vi "StudentScope - PowerSpectrum.vi"(0 "data":dbl[][](array[numeric]), 1 "Cursor Position":dbl, 5 "Acq Rate (Hz)":dbl) -> (14 "Cursor Freq":string, 15 "Ch0 Amp":string, 16 "Ch1 Amp":string, 17 "Ch0 Freq":string, 18 "Ch1 Freq":string, 19 "Normalized Power Spectrum":cluster{"df":dbl, "df":dbl, "Y":dbl[]}[](array[cluster]))   [LabVIEW 2015]
uses:
  <vilib>/measure/matone.llb/Extract Single Tone Information 1 Chan.vi
  <vilib>/Analysis/NI_AALPro.lvlib
  <vilib>/measure/NI_MAPro.lvlib
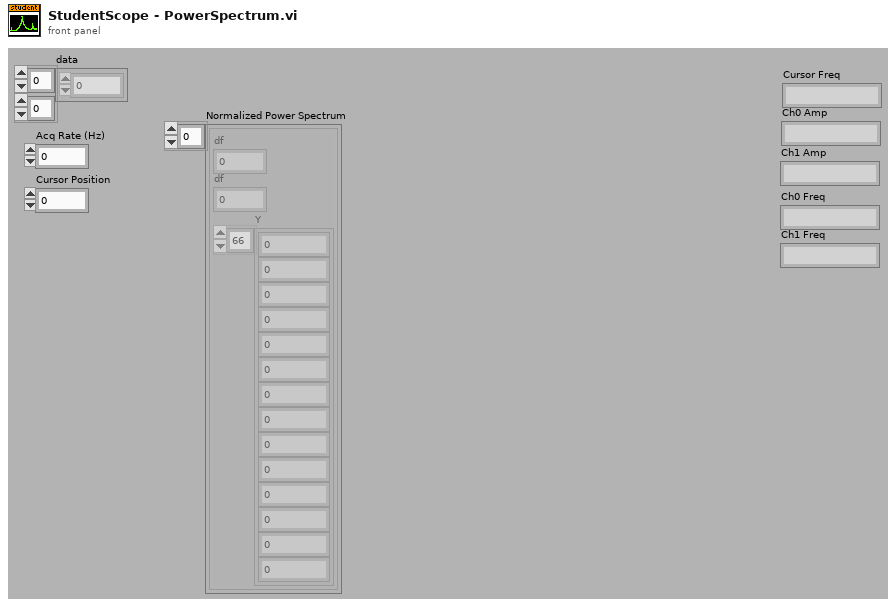
[diagram p1: front panel]
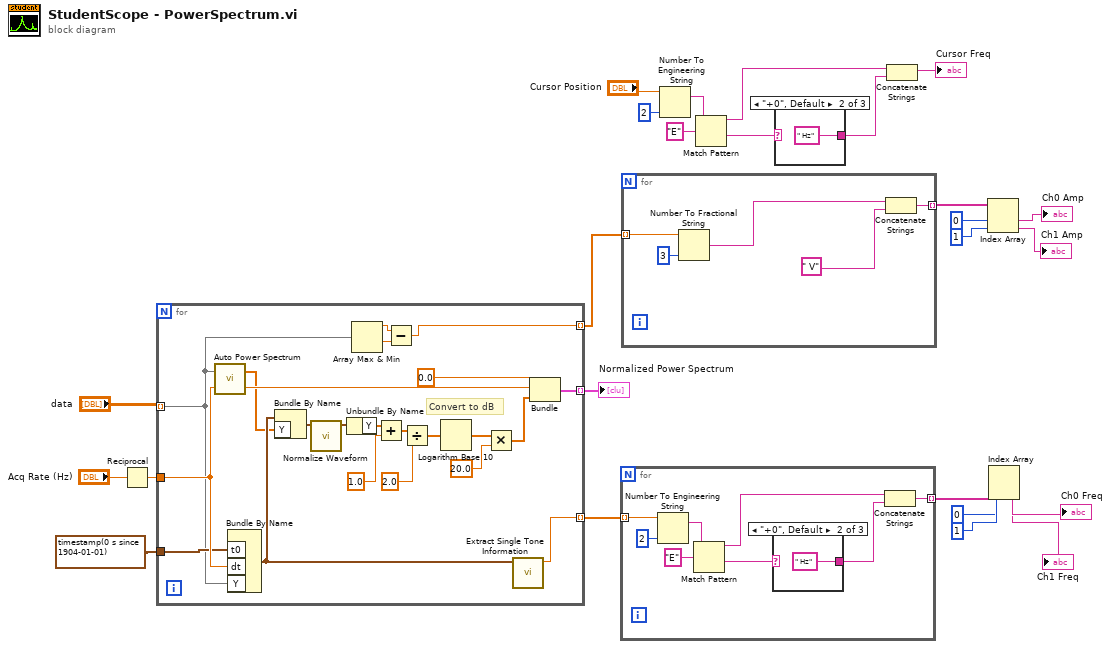
[diagram p0: block diagram]
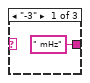
[diagram p2: hidden frame]
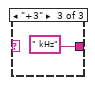
[diagram p3: hidden frame]
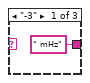
[diagram p4: hidden frame]
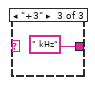
[diagram p5: hidden frame]
diagram:
  n1 = Reciprocal(x="Acq Rate (Hz)") -> (1/x=w23:dbl)
  n2 = for {
    tunnel: "data" -> [w38] mode=indexing
    tunnel: w23 -> [w45]
    tunnel: [w47] -> w20 mode=indexing
    tunnel: [w40] -> w25 mode=indexing
    tunnel: timestamp(0 s since 1904-01-01) ("current time") -> [w39]
    tunnel: [w35] -> w14 mode=indexing
    # "Convert to dB"
    n3 = call <vilib>:"Auto Power Spectrum.vi"("dt"=w45, "Signal (V)"=w38) -> ("df"=w44:dbl, "Power Spectrum (V^2 rms)"=w41:dbl[])
    n4 = Bundle By Name("t0"=w39, "dt"=w45, "Y"=w38) -> (w42:waveform(dbl))  [unwired: 1 in]
    n5 = Bundle By Name(cluster=w42, "Y"=w41) -> (w43:waveform(dbl))
    n6 = call <vilib>:"Normalize Waveform.vi"("waveform in"=w43) -> ("normalized waveform"=w34:waveform(dbl))  [unwired: 7 in, 3 out]
    n7 = Unbundle By Name(w34) -> ("Y"=w31:dbl[])
    n8 = Array Max & Min(array=w38) -> (max value=w37:dbl, min value=w36:dbl)  [unwired: 2 out]
    n9 = Add(x=w31, y=1.0) -> (x+y=w33:dbl[])
    n10 = Subtract(x=w37, y=w36) -> (x-y=w35:dbl)
    n11 = Divide(x=w33, y=2.0) -> (x/y=w27:dbl[])
    n12 = Logarithm Base 10(1:w27) -> (0:w29:dbl[])
    n13 = Multiply(x=w29, y=20.0) -> (x*y=w26:dbl[])
    n14 = call-poly <vilib>:"Extract Single Tone Information.vi"("time signal in"=w42) -> ("detected frequency"=w47:dbl)  [unwired: 5 in, 5 out]
    n15 = Bundle("df"=0.0, "df"=w44, w26) -> (w40:cluster{"df":dbl, "df":dbl, dbl[]})  [unwired: 1 in]
  }
  "Normalized Power Spectrum" <- w25
  n16 = for {
    tunnel: [w49] -> w17 mode=indexing
    tunnel: w20 -> [w48] mode=indexing
    n17 = Number To Engineering String(2:i16 2 ("precision (6)"), 4:w48) -> (0:w55:string)  [unwired: 2 in]
    n18 = Match Pattern(string=w55, regular expression="E" ("string")) -> (before substring=w51:string, after substring=w52:string)  [unwired: 1 in, 2 out]
    n19 = case shown="\"+0\", Default" w52 {
      tunnel: [" mHz" ("string") " Hz" ("string") " kHz" ("string")] -> w50
      frame "-3" {
      }
      frame "+0", Default {
      }
      frame "+3" {
      }
    }
    n20 = Concatenate Strings(w51, w50) -> (w49:string)
  }
  n21 = for {
    tunnel: [w62] -> w11 mode=indexing
    tunnel: w14 -> [w60] mode=indexing
    n22 = Number To Fractional String(number=w60, precision (6)=i16 3) -> (F-format string=w59:string)  [unwired: 2 in]
    n23 = Concatenate Strings(w59, " V" ("string")) -> (w62:string)
  }
  n24 = Number To Engineering String(2:i16 2 ("precision (6)"), 4:"Cursor Position") -> (0:w4:string)  [unwired: 2 in]
  n25 = Match Pattern(string=w4, regular expression="E" ("string")) -> (before substring=w8:string, after substring=w7:string)  [unwired: 1 in, 2 out]
  n26 = case shown="\"+0\", Default" w7 {
    tunnel: [" mHz" ("string") " Hz" ("string") " kHz" ("string")] -> w1
    frame "-3" {
    }
    frame "+0", Default {
    }
    frame "+3" {
    }
  }
  n27 = Concatenate Strings(w8, w1) -> (→"Cursor Freq":string)
  n28 = Index Array(array=w11, index #1=0 ("index"), index #2=1 ("index")) -> (element #1=→"Ch0 Amp":string, element #2=→"Ch1 Amp":string)
  n29 = Index Array(array=w17, index #1=0 ("index"), index #2=1 ("index")) -> (element #1=→"Ch0 Freq":string, element #2=→"Ch1 Freq":string)
